vi "Disabled.vi"(7 "Robot Mode":T2, 10 "Match Info":T1={"Autonomous Elapsed Seconds"=0.0, "TeleOp Elapsed Seconds"=0.0, "Disabled Elapsed Seconds"=0.0, "Visited Autonomous"=FALSE, "Visited TeleOp"=FALSE, "Visited Disabled"=FALSE, "Autonomous Settings"={"Autonomous Style"=enum."Independent", "VI Refnum"=refnum}}, 11 "Call Context":T3) -> ()   [LabVIEW 2018]
doc: "This VI is called each time a disabled packet is received from the DS. It can be used to prepare for the next robot mode, to calibrate sensors, etc."
uses:
  <vilib>/Rock Robotics/WPI/DriverStation/WPI_DriverStationDerivedRobotMode.ctl
  <vilib>/Rock Robotics/WPI/DriverStation/WPI_DriverStationRobotMode2.ctl
  <vilib>/Rock Robotics/WPI/DriverStation/WPI_DriverStationMatch Info.ctl
  <vilib>/Rock Robotics/Network Tables/NT Read String.vi
  <vilib>/Rock Robotics/WPI/Utilities/WPI_GetSetVariantRefNum.vi
  Auton/Command Parser/Active Command.vi
  <vilib>/Rock Robotics/Network Tables/NT Write String Array.vi
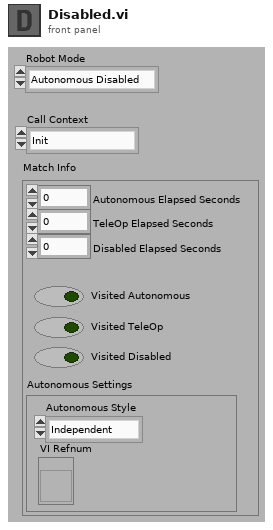
[diagram p1: front panel]
types:
  T1 = typedef "WPI_DriverStationMatch Info.ctl" = cluster{"Autonomous Elapsed Seconds":dbl, "TeleOp Elapsed Seconds":dbl, "Disabled Elapsed Seconds":dbl, "Visited Autonomous":bool, "Visited TeleOp":bool, "Visited Disabled":bool, "Autonomous Settings":cluster{"Autonomous Style":enum16{"Iterative", "Independent"}, "VI Refnum":refnum<vi>}}
  T2 = typedef "WPI_DriverStationRobotMode2.ctl" = enum16{"Autonomous Disabled", "Autonomous Enabled", "Teleop Disabled", "Teleop Enabled", "Disconnected", "Finish", "Test Disabled", "Test Enabled", "Emergency Stopped"}
  T3 = typedef "WPI_DriverStationDerivedRobotMode.ctl" = enum16{"Init", "Execute", "Stop"}
  T4 = typedef "WPI_JoystickDevRef.ctl" = cluster{"Device":T5}
  T5 = typedef "WPI_JoystickDeviceEnum.ctl" = enum16{"USB 0", "USB 1", "USB 2", "USB 3", "USB 4", "USB 5"}
  T6 = typedef "Single Sequence.ctl" = cluster{"Sequence Array":T7[]}
  T7 = typedef "Sequence Command.ctl" = cluster{"Sequence Name":string, "Plate Arrangement":T8, "Command Name":string, "Data":variant, "Sequence Number":u32}
  T8 = typedef "Plate Arrangement.ctl" = cluster{"LR*":bool, "LL*":bool, "RL*":bool, "RR*":bool}
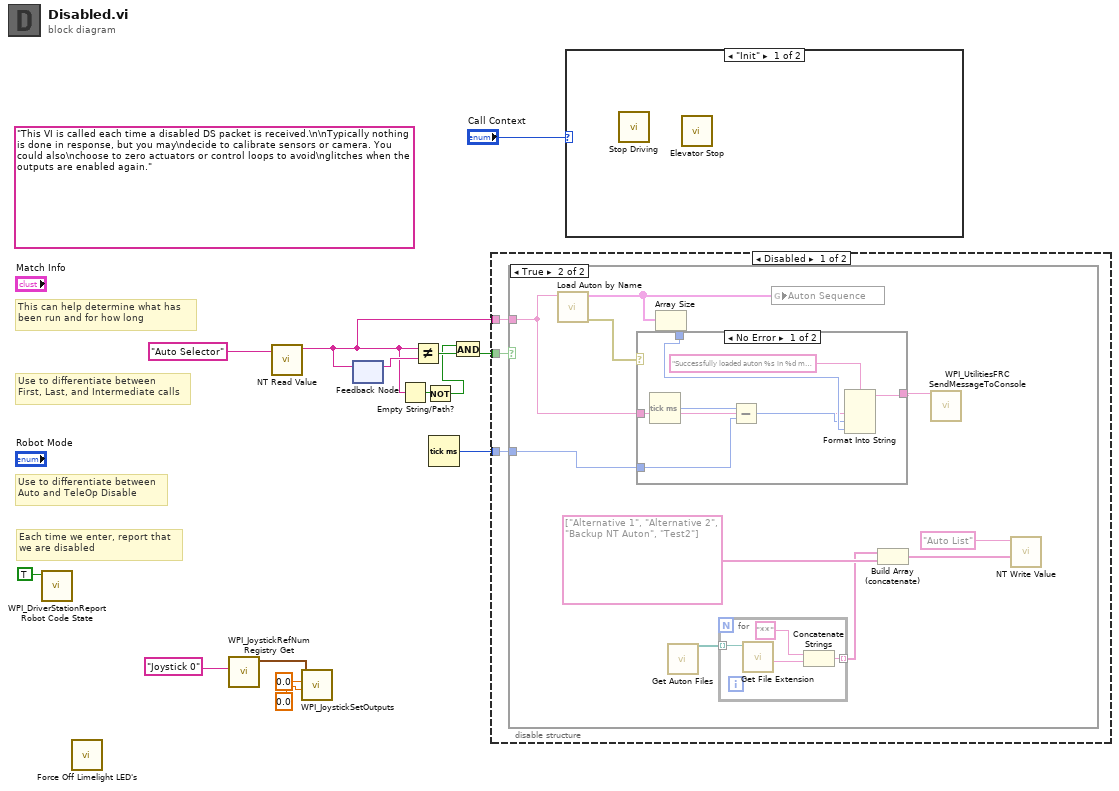
[diagram p0: block diagram]
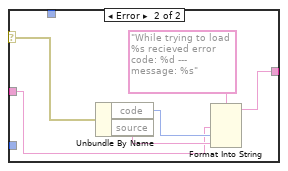
[diagram p3: hidden frame]
diagram:
  (unwired) "This VI is called each time a disabled DS packet is received.\n\nTypically nothing is done in response, but you may\ndecide to calibrate sensors or camera. You could also\nchoose to zero actuators or control loops to avoid\nglitches when the outputs are enabled again."
  # "Each time we enter, report that\nwe are disabled"
  # "Use to differentiate between\nFirst, Last, and Intermediate calls"
  # "This can help determine what has\nbeen run and for how long"
  # "Use to differentiate between\nAuto and TeleOp Disable"
  n1 = call <vilib>:"WPI_DriverStationReport Robot Code State.vi"("Disabled"=TRUE ("Autonomous")) -> ()  [unwired: 10 in, 1 out]
  n2 = call "Force Off Limelight LED's.vi"() -> ()  [unwired: 10 in, 1 out]
  n3 = call <vilib>:"WPI_JoystickRefNum Registry Get.vi"("refnum name"="Joystick 0") -> ("JoystickDevRef"=w1:T4)  [unwired: 1 in, 9 out]
  n4 = call-poly <vilib>:"NT Read Value.vi"("Name"="Auto Selector") -> ("String"=w8:string)  [unwired: 9 in, 1 out]
  n5 = call <vilib>:"WPI_JoystickSetOutputs.vi"("Right Rumble"=sgl 0.0, "Left Rumble"=sgl 0.0, "JoystickDevRef"=w1) -> ()  [unwired: 7 in, 2 out]
  n6 = feedback-in #1(w8) -> ()
  n7 = feedback #1() -> (w12:string)  [unwired: 1 in]
  n8 = Empty String/Path?(string/path=w8) -> (empty?=w7:bool)
  n9 = Not Equal?(x=w8, y=w12) -> (x != y?=w11:bool)
  n10 = Not(x=w7) -> (.not. x?=w6:bool)
  n11 = Tick Count (ms)() -> (millisecond timer value=w10:u32)
  n12 = And(x=w6, y=w11) -> (x .and. y?=w9:bool)
  n13 = disable-structure shown="Disabled" {
    disable-tunnel: w10 -> [w17 _]
    disable-tunnel: w9 -> [w16 _]
    disable-tunnel: w8 -> [w15 _]
    frame Disabled {
      n14 = case shown="True" w16 {
        tunnel: w17 -> [_ w27]
        tunnel: w15 -> [_ w24]
        frame False {
        }
        frame True {
          n15 = call "Load Auton by Name.vi"("String"=w24) -> ("error out"=w28:errorcluster, "Auton Sequence"=w26:T6[])  [unwired: 9 in]
          n16 = Array Size(array=w26) -> (size(s)=w25:i32)
          n17 = case shown="No Error" w28 {
            selector: w28 -> [_ w45]
            tunnel: w27 -> [w38 _]
            tunnel: w25 -> [w36 _]
            tunnel: w24 -> [w34 w41]
            tunnel: [w33 w40] -> w23
            frame No Error {
              n18 = Tick Count (ms)() -> (millisecond timer value=w39:u32)
              n19 = Subtract(x=w39, y=w38) -> (x-y=w35:u32)
              n20 = Format Into String(format string="Successfully loaded auton %s in %d ms with %d sequences.", w34, w35, w36) -> (resulting string=w33:string)  [unwired: 2 in, 1 out]
            }
            frame Error {
              n21 = Unbundle By Name(w45) -> ("code"=w43:i32, "source"=w42:string)
              n22 = Format Into String(format string="While trying to load %s recieved error code: %d --- message: %s", w41, w43, w42) -> (resulting string=w40:string)  [unwired: 2 in, 1 out]
            }
          }
          n23 = call "Get Auton Files.vi"() -> ("All Files in Dir"=w20:path[])  [unwired: 11 in]
          n24 = for {
            tunnel: w20 -> [w32] mode=indexing
            tunnel: [w29] -> w19 mode=indexing
            n25 = call <vilib>:"Get File Extension.vi"("file"=w32) -> ("filename without extension"=w31:string)  [unwired: 6 in, 4 out]
            n26 = Concatenate Strings("**" ("string"), w31) -> (w29:string)
          }
          n27 = global write "Active Command.vi" "Auton Sequence"(w26) -> ()
          n28 = Build Array (concatenate)(w19, string[] ["Alternative 1", "Alternative 2", "Backup NT Auton", "Test2"] ("String Array")) -> (w18:string[])
          n29 = call <vilib>:"WPI_UtilitiesFRC SendMessageToConsole.vi"("Message"=w23) -> ()  [unwired: 14 in, 1 out]
          n30 = call-poly <vilib>:"NT Write Value.vi"("String Array"=w18, "Name"="Auto List") -> ()  [unwired: 9 in, 1 out]
        }
      }
    }
    frame Enabled {
    }
  }
  n31 = case shown="\"Init\"" "Call Context" {
    frame "Init" {
      n32 = call "Stop Driving.vi"() -> ()  [unwired: 11 in, 1 out]
      n33 = call "Elevator Stop.vi"() -> ()  [unwired: 11 in, 1 out]
    }
    frame "Execute", Default {
    }
  }
